vi "Handle Error.vi"(8 "error in (no error)":errorcluster, 11 "Error Handler in":refnum<class "Error Handler.lvclass">) -> (0 "error out":errorcluster, 2 "stop actor?":bool=TRUE, 3 "Error Handler out":refnum<class "Error Handler.lvclass">)   [LabVIEW 2017, in "Error Handler.lvlib" / "Error Handler.lvclass"]
doc: "(<B>Filename</B>: Actor Framework.lvlib:Actor.lvclass:Handle Error.vi)\n\nDefines how the actor handles an error that occurred while processing a message. By default, this method does nothing except stop the actor."
uses:
  Error Handler.lvclass
  <vilib>/ActorFramework/Actor/Actor.lvclass
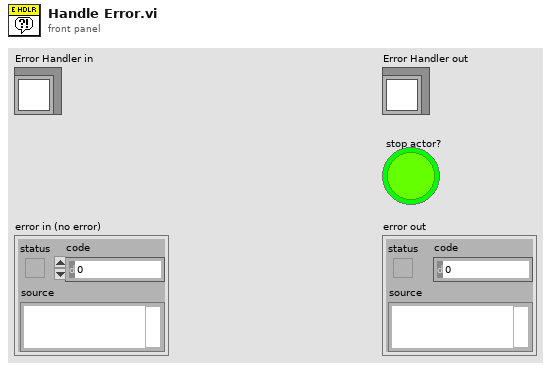
[diagram p1: front panel]
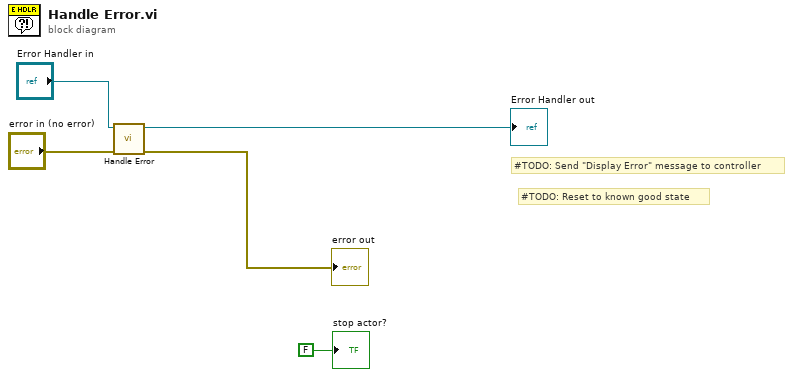
[diagram p0: block diagram]
diagram:
  # "#TODO: Reset to known good state"
  # "#TODO: Send \"Display Error\" message to controller"
  n1 = call-parent "Handle Error.vi"("error in (no error)"="error in (no error)", "Actor in"="Error Handler in") -> ("error out"=→"error out":errorcluster, "Actor out"=→"Error Handler out":refnum<class "Error Handler.lvclass">)  [unwired: 7 in, 1 out]
  "stop actor?" <- FALSE
